vi "Translator.File.Write.vi"(8 "error in":errorcluster, 10 "Language in use":string, 11 "Translation folder":path=path "D:/PL_0125_Sapphire_Automation/settings") -> (0 "error out":errorcluster)   [LabVIEW 2015]
uses:
  Translator.Enums.ctl
  Translator.Message.ctl
  EventLog/EventLog.EventLevelGui.ctl
  Windows/Windows.ExitAction.ctl
  TouchPanel/TouchPanelMonths.ctl
  EventLog/EventLog.EventSource.ctl
  Sequence/Sequence.Step.Status.ctl
  Sequence/Sequence.MainMode.ctl
  Gui/ResultsGui.IncludeOptions.ctl
  <vilib>/Utility/config.llb/Read Key (String).vi
  <vilib>/Utility/config.llb/Write Key (String).vi
  <vilib>/Utility/config.llb/NI_LVConfig.lvlib
panel:
  in  "Enums":T1={"Msg"=enum."-", "Level"=enum."Debug", "ExitAction"=enum."Log off from PC", "Month"=enum."February", "Source"=enum."Gui", "TestStatus"=enum."-", "GuiMode"=enum."Auto", "ResOptions"=enum."All"}
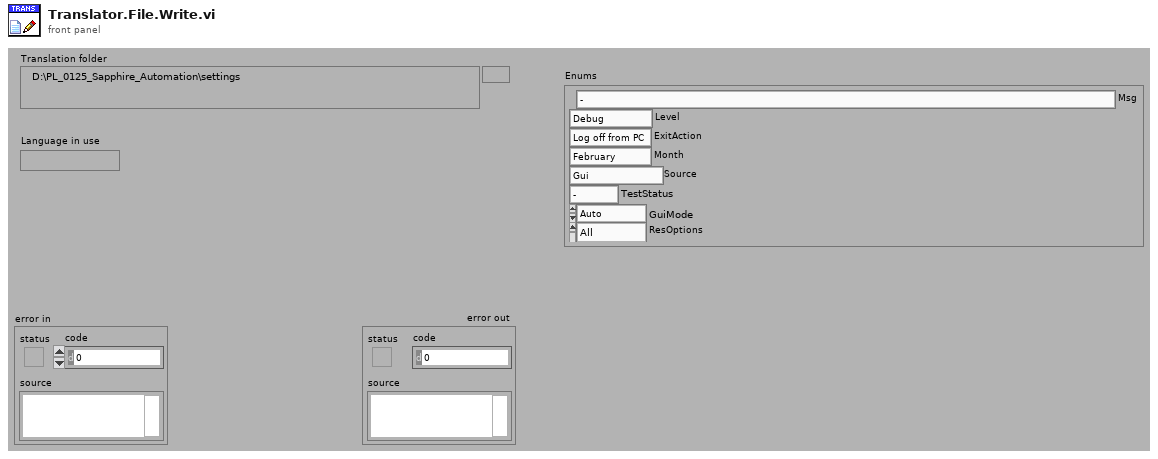
[diagram p1: front panel]
types:
  T1 = typedef "Translator.Enums.ctl" = cluster{"Msg":T2, "Level":T3, "ExitAction":T4, "Month":T5, "Source":T6, "TestStatus":T7, "GuiMode":T8, "ResOptions":T9}
  T2 = typedef "Translator.Message.ctl" = enum16{"-", "Event confirmed", "Log out", "Log in", "Shutdown", "Cancel", "Start", "On", "Off", "OK", "NOK", "NOK %s", "Home", "Work", "Close", "Open", "In progress...", "Missing", "Empty", "Hardware failure", "Initial", "Error %d >> %s", "Error %d >> %s >> %s", "Msg %d >> %s", "Unable to reset Laser Interlock (%s)", "Unable to reset Laser Shutterlock. Laser not ready  (%s)", "Laser marking timeout", "Starting %s", "Quitting %s", "Configured", "Initializing", "Quitting", "Loading", "Running", "Stopped", "Summary", "Laser", "Do you want to continue?", "Press confirm button", "Station is not based. Do you want to exit?", "Station requires changeover. Do you want to run the test?", "Test options are not set as default. Do you want to continue?", "Product not detected. Do you want to continue?", "Product scan failed. Do you want to continue?", "Calibration", "Log out?", "System", "All", "IDLE", "Translating...%s", "Not found", "Alarm %s", "Run", "Skip", "Abort", "Repeat", "Please wait...", "Database disconnected", "Database disconnected - changeover disabled!", "Login to database successful", "Login to database failed: %d; %s", "Unable to check the product status of reference %d - database disconnected", "Unable to set the product status of reference %d - database disconnected", "Variant file backup %s", "Read steps (%s)", "Result", "Station armed!", "Station requires changeover!", "Select reference number...", "EMERGENCY BUTTON - press Control button", "EMERGENCY DOOR - press Control button", "Resetting Emergency...", "Unable to reset safety circuit - Emergency Button pressed", "Unable to reset safety circuit - Emergency Front Door open", "Unable to reset safety circuit - Emergency Side Door open", "Station not based", "Station not empty", "Station basing...", "Unkown reference", "Reference %d missing", "Reference invalid", "Wrong revolver", "Container missing", "Door open", "Close the front door", "Press start button", "Test done. Open the front door", "Test %s", "Test OK", "Test NOK", "Test error - press Confirm button", "Test stopped", "Remove product", "Confirm failure", "Test running...", "Test running... %.1f %%", "Stopping test...", "Finalizing test...", "Sequence folder '%s' is missing", "File '%s' is missing", "File '%s' is broken", "File '%s' is running", "Log file '%s' started", "Step '%s' added to log file", "Step '%s' graph added to log file", "Log file '%s' ended", "Log file '%s' ignored", "Log file '%s' exported", "Log file '%s' export failed", "Wrong serial number in log file", "Wrong reference number in log file", "Test steps are missing", "%s = %.3f", "Process param '%s' not found in DB", "Process param '%s' wrong order", "Process param '%s' value %.3f out of limits (%.3f; %.3f)", "Step%d param '%s' not found in DB", "Step%d param '%s' wrong order", "Step%d param '%s' value %.3f out of limits (%.3f; %.3f)", "Step%d EV '%s' not found in DB", "Step%d EV '%s' wrong order", "\"%s\" not found in DB", "\"%s\" wrong order", "\"%s\" value %.3f out of limits (%.3f; %.3f)", "\"%s\" not found in software", "Sequence initialized (%d)", "Sequence started", "Sequence done", "Sequence aborted", "Sequence aborted at work", "Sequence aborted at home", "Sequence error", "Seqeunce error at home", "Sequence error at work", "Scan failed. Error %s", "Scan failed. Scanner disconnected", "Scan failed. Wrong Wabco number %d, limit (%d,%d)", "Scan failed. Wrong serial number %d, limit (%d,%d)", "Scan failed. Wrong date %d, limit (%d,%d)", "Scan failed. Wrong product wabco number %d (expected %d)", "Scan failed. Wrong product serial number %d (expected > 0)", "Scan OK %s", "%s = %d", "%s = %d->%d", "Unable to set %s = %.2f - Air Pressure Inside off", "Unable to reset Emergency Circuit - emg button", "Unable to reset Emergency Circuit - light curtain", "Unable to reset Emergency Circuit - door open", "Unable to set digital output '%s' = %d", "Unable to activate air pressure inside - timeout", "Unable to activate air pressure inside - aborted", "Unable to switch on Air Main Valve - Air Pressure Inlet off", "Unable to switch on Air Main Valve - Door open", "Unable to switch off Air Main Valve - timeout", "Unable to switch off Air Main Valve - aborted", "Unable to rotate Table - timeout", "Unable to rotate Table - aborted", "Unable to rotate Table - Air Pressure Inside off", "Unable to rotate Table - Product Lift A not in Home position", "Unable to rotate Table - Product Lift B not in Home position", "Unable to rotate Table - unlock before movement timeout", "Unable to rotate Table - lock after movement timeout", "Unable to move Table Lock to %s position - timeout", "Unable to move Table Lock to %s position - aborted", "Unable to move Table Lock to %s position - Air Pressure Inside off", "Unable to move Table Lock to %s position - Table not in position", "Unable to move Product Lift A to %s position - timeout", "Unable to move Product Lift B to %s position - timeout", "Unable to move Product Lift A to %s position - aborted", "Unable to move Product Lift B to %s position - aborted", "Unable to move Product Lift A to %s position - Air Pressure Inside off", "Unable to move Product Lift B to %s position - Air Pressure Inside off", "Unable to move Product Lift A to %s position - Table not locked", "Unable to move Product Lift B to %s position - Table not locked", "Unable to move Product Lift A to %s position - Product Arm not in Work position", "Unable to move Product Lift B to %s position - Product Arm not in Work position", "Unable to set Product Suction Gripper %s to %s - timeout", "Unable to set Product Suction Gripper %s to %s - aborted", "Unable to move Product Arm to %s position - timeout", "Unable to move Product Arm to %s position - aborted", "Unable to move Product Arm to %s position - Air Pressure Inside off", "Unable to move Product Arm to %s position - Product Lift A not in Home position", "Unable to move Product Arm to %s position - Product Lift B not in Home position", "Unable to move Product to %s position - timeout", "Unable to move Product to %s position - aborted", "Unable to move Product to %s position - Air Pressure Inside off", "Unable to move Product to %s position - Table not in position"}
  T3 = typedef "EventLog.EventLevelGui.ctl" = enum16{"ALL", "Debug", "Info", "Warning", "Error"}
  T4 = typedef "Windows.ExitAction.ctl" = enum16{"Log off from PC", "Shut Down PC", "Reboot PC", "Close Program"}
  T5 = typedef "TouchPanelMonths.ctl" = enum16{"January", "February", "March", "April", "May", "June", "July", "August", "September", "October", "November", "December"}
  T6 = typedef "EventLog.EventSource.ctl" = enum16{"All", "Gui", "Ref", "File", "Seq", "Scan", "Lock", "AO", "AI", "CI", "DIO", "CPX", "PS", "Proda", "Trace", "Laser", "Scanner Prod", "Scanner Order"}
  T7 = typedef "Sequence.Step.Status.ctl" = enum16{"-", "Pending", "Running", "Skipped", "Passed", "Failed", "Done", "Error", "Aborted", "Stopped"}
  T8 = typedef "Sequence.MainMode.ctl" = enum16{"Auto", "Step", "Base", "Changeover", "Manual", "Logs", "Results"}
  T9 = typedef "ResultsGui.IncludeOptions.ctl" = enum16{"All", "Temporary", "Exported", "Error"}
  T10 = typedef "NI_LVConfig.lvlib/Config Data RefNum.ctl" = refnum<k1>
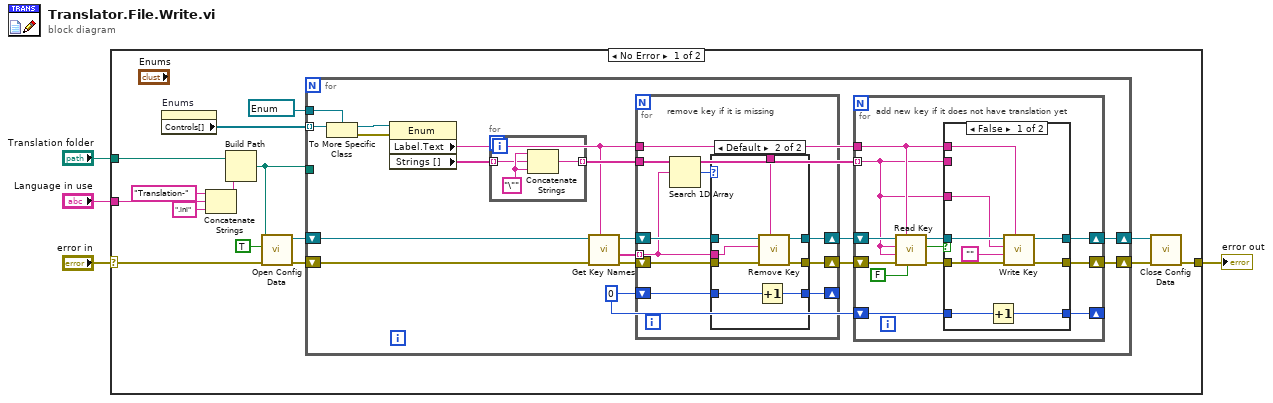
[diagram p0: block diagram]
diagram:
  n1 = case shown="No Error" "error in" {
    selector: "error in" -> [w12 w85]
    tunnel: "Translation folder" -> [w19 _]
    tunnel: [w6 w85] -> w3
    tunnel: "Language in use" -> [w18 _]
    frame No Error {
      n2 = property on="Enums" class="Clust (strict)"() -> ("Controls[]"=w14:refnum<vi>[])  [unwired: 2 in, 2 out]
      n3 = Concatenate Strings("Translation-" ("string"), w18, ".ini" ("string")) -> (w17:string)
      n4 = Build Path(base path=w19, name or relative path=w17) -> (appended path=w11:path)
      n5 = call <vilib>:"Open Config Data.vi"("error in (no error)"=w12, "create file if necessary (T)"=TRUE, "configuration file path"=w11) -> ("error out"=w10:errorcluster, "refnum"=w9:T10)  [unwired: 6 in, 1 out]
      n6 = for {
        shift-right: [w20] -> w7
        shift-left: w10 -> [w29]
        tunnel: w14 -> [w28] mode=indexing
        tunnel: w11 -> [_]
        tunnel: refnum<vi> refnum ("reference out") -> [w25]
        shift-right: [w21] -> w8
        shift-left: w9 -> [w22]
        w31 = 0
        n7 = To More Specific Class(target class=w25, reference=w28) -> (specific class reference=w27:refnum<vi>, error out=w26:errorcluster)  [unwired: 1 in]
        n8 = property class="Enum"(reference=w27, error in=w26) -> ("Label.Text"=w23:string, "Strings []"=w24:string[])  [unwired: 2 out]
        n9 = for {
          tunnel: w24 -> [w38] mode=indexing
          tunnel: [w37] -> w30 mode=indexing
          w39 = "\""
          n10 = Concatenate Strings(w39, w38, w39) -> (w37:string)
        }
        n11 = call <vilib>:"Get Key Names.vi"("section"=w23, "error in (no error)"=w29, "refnum"=w22) -> ("error out"=w36:errorcluster, "key names"=w32:string[], "refnum out"=w33:T10)  [unwired: 5 in, 1 out]
        n12 = for {
          shift-right: [w46] -> w35
          shift-left: w36 -> [w49]
          shift-right: [w48] -> w34
          shift-left: w33 -> [w47]
          tunnel: w32 -> [w44] mode=indexing
          tunnel: w30 -> [w45]
          tunnel: w23 -> [w42]
          shift-right: [w40] -> _
          shift-left: w31 -> [w41]
          # "remove key if it is missing"
          n13 = Search 1D Array(1D array=w45, element=w44) -> (index of element=w43:i32)  [unwired: 1 in]
          n14 = case shown="Default" w43 {
            tunnel: w49 -> [w52 w60]
            tunnel: [w51 w59] -> w48
            tunnel: w47 -> [w51 w58]
            tunnel: w44 -> [_ w57]
            tunnel: [w52 w56] -> w46
            tunnel: w42 -> [_ w55]
            tunnel: w41 -> [w50 w54]
            tunnel: [w50 w53] -> w40
            frame 0.. {
            }
            frame Default {
              n15 = Increment(x=w54) -> (x+1=w53:i32)
              n16 = call <vilib>:"Remove Key.vi"("section"=w55, "error in (no error)"=w60, "key"=w57, "refnum"=w58) -> ("error out"=w56:errorcluster, "refnum out"=w59:T10)  [unwired: 5 in, 1 out]
            }
          }
        }
        n17 = for {
          tunnel: w23 -> [w68]
          tunnel: w30 -> [w61] mode=indexing
          shift-right: [w72] -> w20
          shift-left: w35 -> [w69]
          shift-right: [w71] -> w21
          shift-left: w34 -> [w70]
          shift-right: [w63] -> _
          shift-left: w31 -> [w64]
          # "add new key if it does not have translation yet"
          n18 = call-poly <vilib>:"Read Key.vi"("read raw string? (F)"=FALSE, "section"=w68, "error in (no error)"=w69, "default value"=w61, "key"=w61, "refnum"=w70) -> ("error out"=w65:errorcluster, "found?"=w67:bool, "refnum out"=w66:T10)  [unwired: 2 in, 1 out]
          n19 = case shown="False" w67 {
            tunnel: [w81 w83] -> w72
            tunnel: [w80 w84] -> w71
            tunnel: w66 -> [w79 w84]
            tunnel: w65 -> [w78 w83]
            tunnel: w68 -> [w77 _]
            tunnel: w61 -> [_ _]
            tunnel: [w74 w82] -> w63
            tunnel: w64 -> [w75 w82]
            tunnel: w61 -> [w73 _]
            frame False {
              n20 = Increment(x=w75) -> (x+1=w74:i32)
              n21 = call-poly <vilib>:"Write Key.vi"("section"=w77, "error in (no error)"=w78, "value"="", "key"=w73, "refnum"=w79) -> ("error out"=w81:errorcluster, "refnum out"=w80:T10)  [unwired: 4 in, 1 out]
            }
            frame True {
            }
          }
        }
      }
      n22 = call <vilib>:"Close Config Data.vi"("error in (no error)"=w7, "refnum"=w8) -> ("error out"=w6:errorcluster)  [unwired: 8 in, 1 out]
    }
    frame Error {
    }
  }
  "error out" <- w3
